vi "Tektronix_measure_3ch.vi"(8 "error in (no error)":errorcluster, 11 "VISA resource name":refnum<visa-resource-name>="USB0::0x0699::0x03B3::C020727::INSTR") -> (0 "error out":errorcluster, 1 "Measurement 2":dbl, 2 "Measurement 1":dbl, 3 "VISA resource name out":refnum<visa-resource-name>, 4 "read buffer 2":string, 5 "read buffer 1":string, 6 "Measurement 3":dbl, 7 "read buffer 3":string)   [LabVIEW 2017]
panel:
  out "remaining string":string
  in  "CH2 Range (V)":string="5.0"
  in  "CH1 Range (V)":string="5.0"
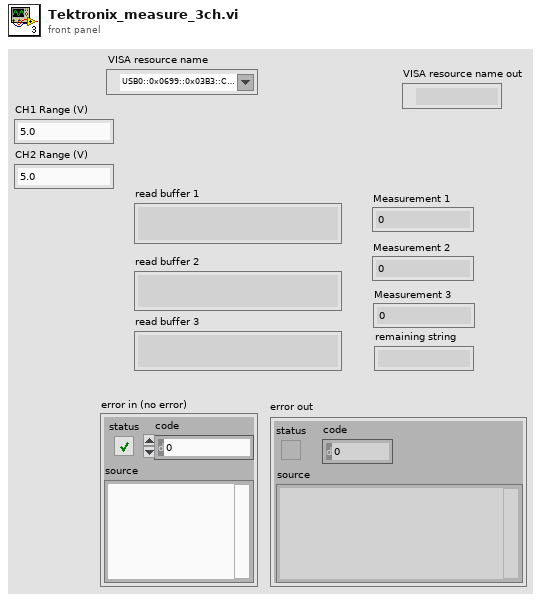
[diagram p1: front panel]
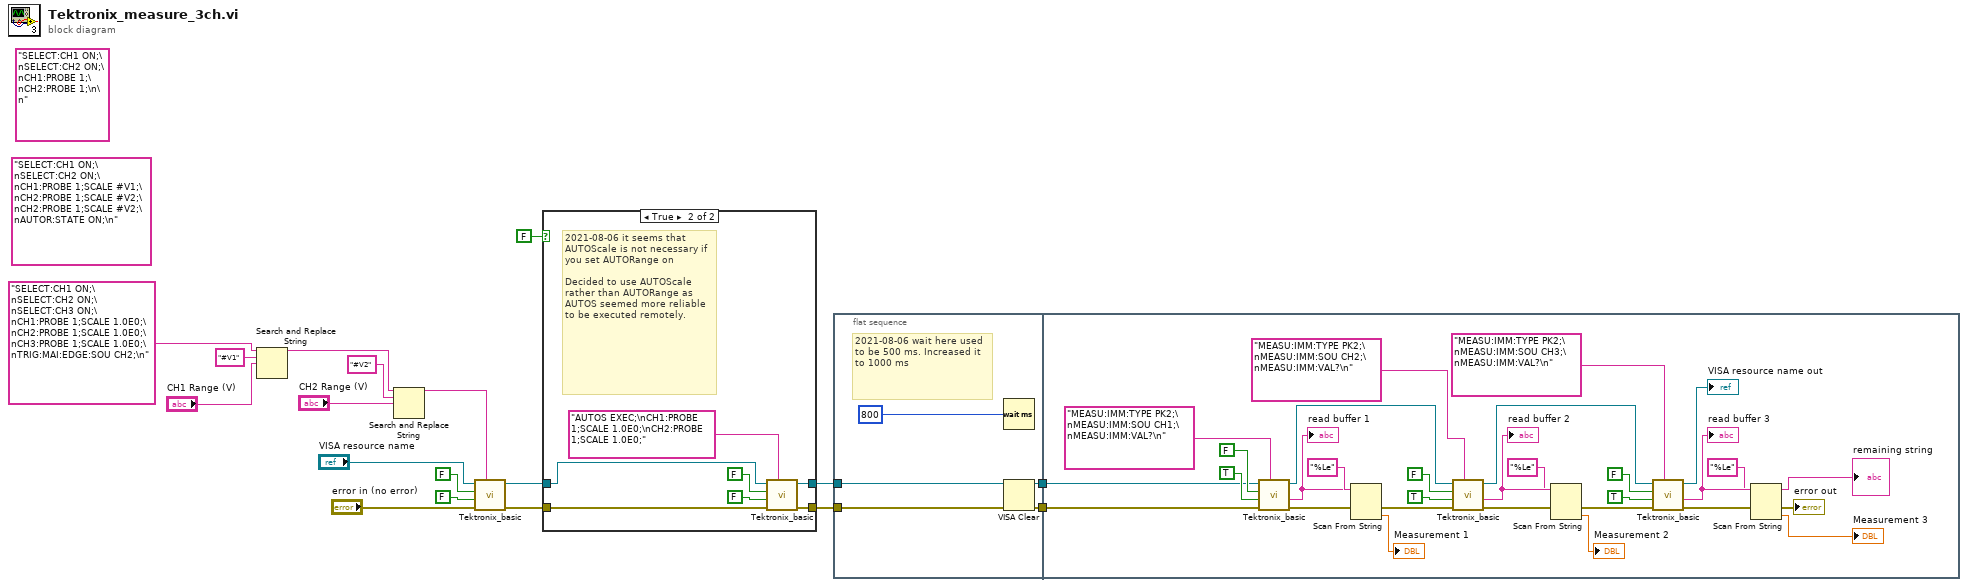
[diagram p0: block diagram]
diagram:
  (unwired) "SELECT:CH1 ON;\nSELECT:CH2 ON;\nCH1:PROBE 1;SCALE #V1;\nCH2:PROBE 1;SCALE #V2;\nCH2:PROBE 1;SCALE #V2;\nAUTOR:STATE ON;\n" ("write buffer")
  (unwired) "SELECT:CH1 ON;\nSELECT:CH2 ON;\nCH1:PROBE 1;\nCH2:PROBE 1;\n\n" ("write buffer")
  n1 = Search and Replace String(input string="SELECT:CH1 ON;\nSELECT:CH2 ON;\nSELECT:CH3 ON;\nCH1:PROBE 1;SCALE 1.0E0;\nCH2:PROBE 1;SCALE 1.0E0;\nCH3:PROBE 1;SCALE 1.0E0;\nTRIG:MAI:EDGE:SOU CH2;\n" ("write buffer"), search string="#V1", replace string="CH1 Range (V)") -> (result string=w7:string)  [unwired: 5 in, 3 out]
  n2 = Search and Replace String(input string=w7, search string="#V2", replace string="CH2 Range (V)") -> (result string=w6:string)  [unwired: 5 in, 3 out]
  n3 = call "Tektronix_basic.vi"("write buffer"=w6, "error in (no error)"="error in (no error)", "Query?"=FALSE, "Error query?"=FALSE, "VISA resource name"="VISA resource name") -> ("error out"=w13:errorcluster, "VISA resource name out"=w14:refnum<visa-resource-name>)  [unwired: 4 in, 1 out]
  n4 = case shown="TRUE" FALSE {
    tunnel: w14 -> [w20 w25]
    tunnel: w13 -> [w19 w24]
    tunnel: [w19 w23] -> w12
    tunnel: [w20 w22] -> w11
    frame False {
    }
    frame True {
      # "2021-08-06 it seems that AUTOScale is not necessary if you set AUTORange on\n\nDecided to use AUTOScale rather than AUTORange as  AUTOS seemed more reliable to be executed remotely."
      n5 = call "Tektronix_basic.vi"("write buffer"="AUTOS EXEC;\nCH1:PROBE 1;SCALE 1.0E0;\nCH2:PROBE 1;SCALE 1.0E0;", "error in (no error)"=w24, "Query?"=FALSE, "Error query?"=FALSE, "VISA resource name"=w25) -> ("error out"=w23:errorcluster, "VISA resource name out"=w22:refnum<visa-resource-name>)  [unwired: 4 in, 1 out]
    }
  }
  n6 = flat-sequence {
    tunnel: w11 -> [w32]
    tunnel: w12 -> [w31]
    tunnel: [w30] -> w10
    tunnel: [w29] -> w8
    tunnel: w10 -> [w60]
    tunnel: w8 -> [w59]
    frame #0 {
      # "2021-08-06 wait here used to be 500 ms. Increased it to 1000 ms"
      n7 = Wait (ms)(milliseconds to wait=u32 800) -> ()  [unwired: 1 out]
      n8 = VISA Clear(VISA resource name=w32, error in (no error)=w31) -> (VISA resource name out=w29:refnum<visa-resource-name>, error out=w30:errorcluster)
    }
    frame #1 {
      n9 = call "Tektronix_basic.vi"("write buffer"="MEASU:IMM:TYPE PK2;\nMEASU:IMM:SOU CH1;\nMEASU:IMM:VAL?\n", "error in (no error)"=w60, "Query?"=TRUE, "Error query?"=FALSE, "VISA resource name"=w59) -> ("error out"=w48:errorcluster, "read buffer"=w52:string, "VISA resource name out"=w45:refnum<visa-resource-name>)  [unwired: 4 in]
      "read buffer 1" <- w52
      n10 = Scan From String(format string="%Le", input string=w52, error in=w48) -> (error out=w46:errorcluster, output 1=→"Measurement 1":dbl)  [unwired: 2 in, 2 out]
      n11 = call "Tektronix_basic.vi"("write buffer"="MEASU:IMM:TYPE PK2;\nMEASU:IMM:SOU CH2;\nMEASU:IMM:VAL?\n", "error in (no error)"=w46, "Query?"=TRUE, "Error query?"=FALSE, "VISA resource name"=w45) -> ("error out"=w56:errorcluster, "read buffer"=w58:string, "VISA resource name out"=w41:refnum<visa-resource-name>)  [unwired: 4 in]
      "read buffer 2" <- w58
      n12 = Scan From String(format string="%Le", input string=w58, error in=w56) -> (error out=w38:errorcluster, output 1=→"Measurement 2":dbl)  [unwired: 2 in, 2 out]
      n13 = call "Tektronix_basic.vi"("write buffer"="MEASU:IMM:TYPE PK2;\nMEASU:IMM:SOU CH3;\nMEASU:IMM:VAL?\n", "error in (no error)"=w38, "Query?"=TRUE, "Error query?"=FALSE, "VISA resource name"=w41) -> ("error out"=w44:errorcluster, "read buffer"=w35:string, "VISA resource name out"=→"VISA resource name out":refnum<visa-resource-name>)  [unwired: 4 in]
      "read buffer 3" <- w35
      n14 = Scan From String(format string="%Le" ("形式文字列"), input string=w35, error in=w44) -> (remaining string=→"remaining string":string, error out=→"error out":errorcluster, output 1=→"Measurement 3":dbl)  [unwired: 1 in, 2 out]
    }
  }
